vi "State Processing Logic.vi"(8 "error in":errorcluster, 9 "State":T1, 10 "Parameter":variant, 11 "User Input":T2 caption="Command") -> (0 "error out":errorcluster, 2 "Feedback":variant caption="Parameter", 3 "State Out":T1 caption="State")   [LabVIEW 2011]
doc: "[Covers: AB3]\n[Covers: AB4]"
uses:
  TypeDefs/UI to CTRL Command.ctl
  TypeDefs/ATM Controller State.ctl
  TypeDefs/Simulated Database Command.ctl
  TypeDefs/User Console Commands.ctl
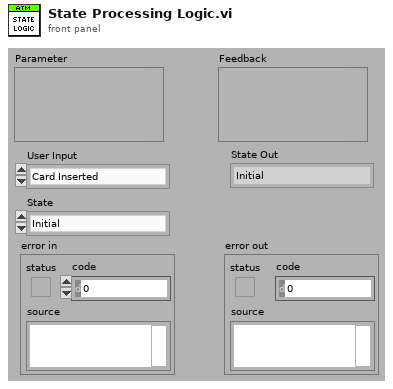
[diagram p1: front panel]
types:
  T1 = typedef "ATM Controller State.ctl" = enum16{"Initial", "Login", "Main Menu", "Balance Inquiry", "Deposit", "Deposit Complete", "Withdrawal", "Withdrawal Success", "Withdrawal Failure", "Terminate", "Lock Out"}
  T2 = typedef "UI to CTRL Command.ctl" = enum16{"Card Inserted", "Keypad Entry", "Button Pressed"}
  T3 = typedef "Simulated Database Command.ctl" = enum16{"Init", "Look up and Lock Account", "Modify Balance", "Get Record", "Commit Record", "Unlock Record", "Close"}
  T4 = typedef "User Console Commands.ctl" = enum16{"Init", "Set ATM Message", "Set ATM Menus", "Disable Controls", "Wait for Input", "Clear Keypad", "Return Card", "Close"}
  T5 = enum16{"Init", "Handle", "Check", "Close", "Set Current Account"}
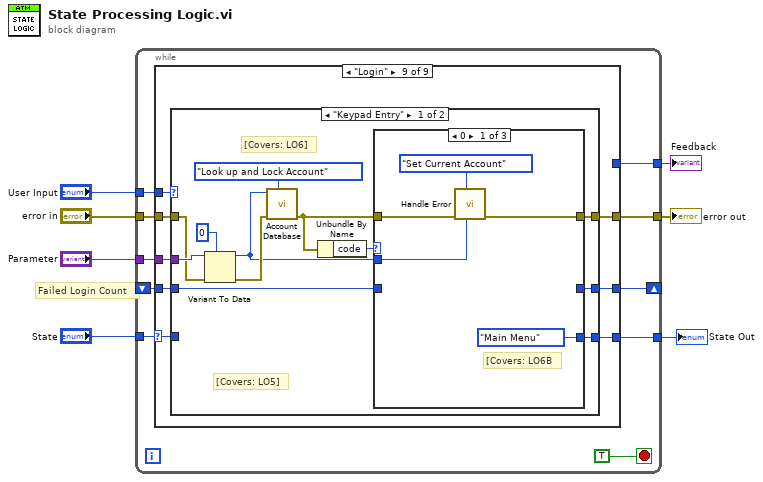
[diagram p0: block diagram]
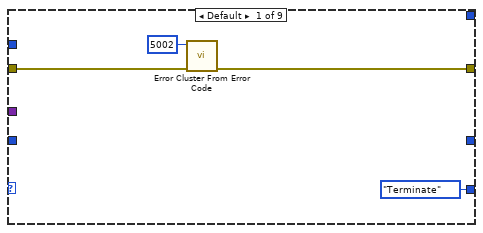
[diagram p2: hidden frame]
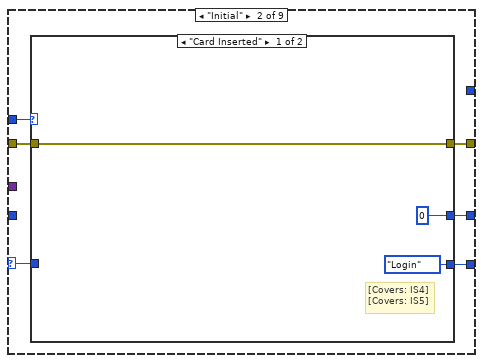
[diagram p3: hidden frame]
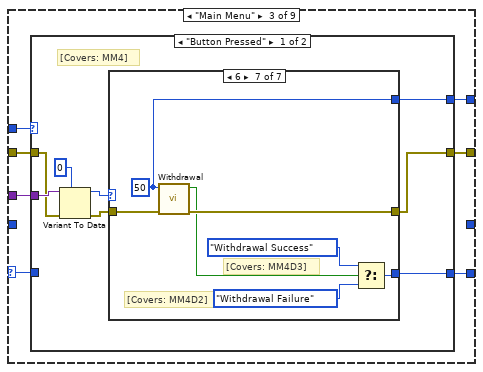
[diagram p5: hidden frame]
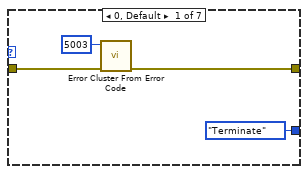
[diagram p6: hidden frame]
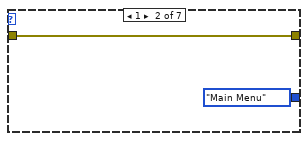
[diagram p7: hidden frame]
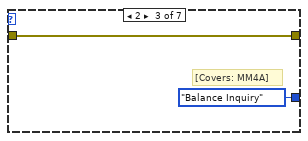
[diagram p8: hidden frame]
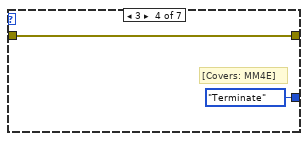
[diagram p9: hidden frame]
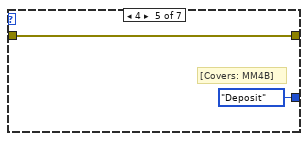
[diagram p10: hidden frame]
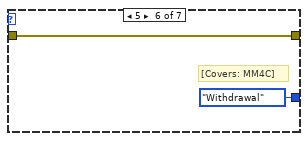
[diagram p11: hidden frame]
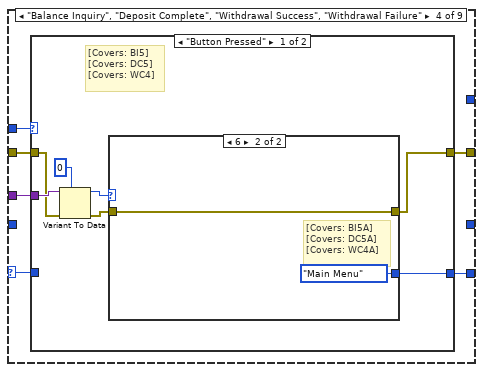
[diagram p13: hidden frame]
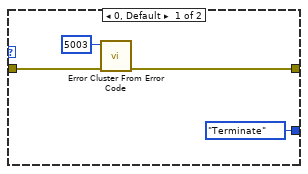
[diagram p14: hidden frame]
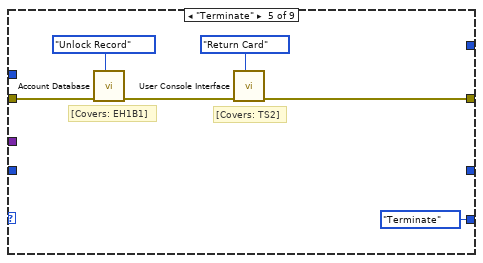
[diagram p16: hidden frame]
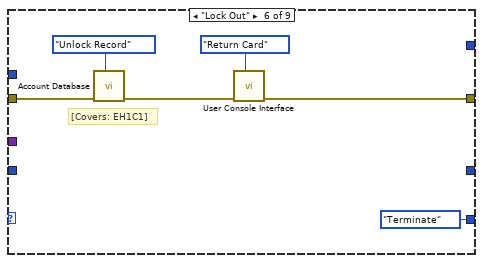
[diagram p17: hidden frame]
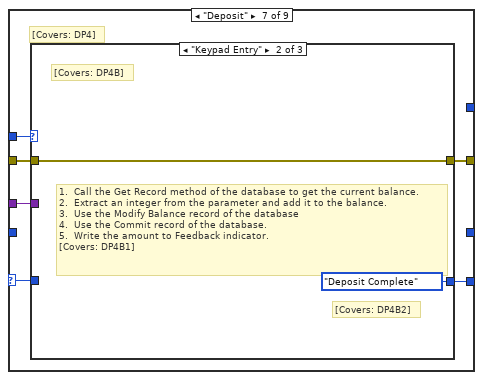
[diagram p18: hidden frame]
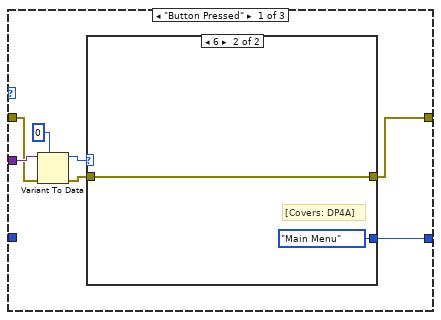
[diagram p19: hidden frame]
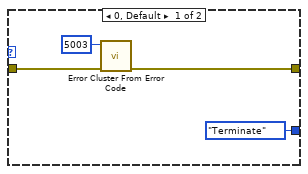
[diagram p20: hidden frame]
diagram:
  # "Failed Login Count"
  n1 = while {
    tunnel: [w17] -> w7
    tunnel: "error in" -> [w16]
    tunnel: "User Input" -> [w15]
    tunnel: "State" -> [w14]
    tunnel: [w13] -> w3
    tunnel: "Parameter" -> [w12]
    shift-right: [w10] -> _
    shift-left: _ -> [w9]
    tunnel: [w8] -> w1
    stop <- TRUE stop-if-true
    n2 = case shown="\"Login\"" w14 {
      selector: w14 -> [_ w23 w35 w72 _ _ w105 w129 w162]
      tunnel: w15 -> [_ w27 w39 w76 _ _ w109 w133 w166]
      tunnel: w16 -> [w20 w26 w38 w75 w94 w100 w108 w132 w165]
      tunnel: [w18 w25 w37 w74 w95 w101 w107 w131 w164] -> w17
      tunnel: [ATM_Controller_State."Terminate" ("State") w24 w36 w73 ATM_Controller_State."Terminate" ("State") ATM_Controller_State."Terminate" ("State") w106 w130 w163] -> w13
      tunnel: w12 -> [_ _ w34 w71 _ _ w104 w128 w161]
      tunnel: [_ w22 _ _ _ _ _ _ w159] -> w10
      tunnel: w9 -> [_ _ _ _ _ _ _ _ w160]
      tunnel: [_ _ w33 _ _ _ _ w127 _] -> w8
      frame Default {
        n3 = call <vilib>:"Error Cluster From Error Code.vi"("error in (no error)"=w20, "error code (0)"=5002) -> ("error out"=w18:errorcluster)  [unwired: 7 in]
      }
      frame "Initial" {
        n4 = case shown="\"Card Inserted\"" w27 {
          tunnel: w26 -> [w29 w32]
          tunnel: [w29 w32] -> w25
          tunnel: [ATM_Controller_State."Login" ("State Out") w31] -> w24
          tunnel: w23 -> [_ w31]
          tunnel: [0 _] -> w22
          frame "Card Inserted" {
            # "[Covers: IS4]\n[Covers: IS5]"
          }
          frame Default {
          }
        }
      }
      frame "Main Menu" {
        n5 = case shown="\"Button Pressed\"" w39 {
          tunnel: w38 -> [w46 w70]
          tunnel: [w42 w70] -> w37
          tunnel: [w41 w69] -> w36
          tunnel: w35 -> [_ w69]
          tunnel: w34 -> [w47 _]
          tunnel: [w40 _] -> w33
          frame "Button Pressed" {
            # "[Covers: MM4]"
            n6 = Variant To Data(error in=w46, type=0 ("index"), Variant=w47) -> (data=w44:i32, error out=w43:errorcluster)
            n7 = case shown="6" w44 {
              tunnel: w43 -> [w51 w53 w55 w57 w59 w61 w68]
              tunnel: [w49 w53 w55 w57 w59 w61 w67] -> w42
              tunnel: [ATM_Controller_State."Terminate" ("State") ATM_Controller_State."Main Menu" ("State") ATM_Controller_State."Balance Inquiry" ("State") ATM_Controller_State."Terminate" ("State") ATM_Controller_State."Deposit" ("State") ATM_Controller_State."Withdrawal" ("State") w63] -> w41
              tunnel: [_ _ _ _ _ _ w62] -> w40
              frame 0, Default {
                n8 = call <vilib>:"Error Cluster From Error Code.vi"("error in (no error)"=w51, "error code (0)"=5003) -> ("error out"=w49:errorcluster)  [unwired: 7 in]
              }
              frame 1 {
              }
              frame 2 {
                # "[Covers: MM4A]"
              }
              frame 3 {
                # "[Covers: MM4E]"
              }
              frame 4 {
                # "[Covers: MM4B]"
              }
              frame 5 {
                # "[Covers: MM4C]"
              }
              frame 6 {
                w62 = 50 ("Amount")
                # "[Covers: MM4D3]"
                # "[Covers: MM4D2]"
                n9 = call "Withdrawal.vi"("error in (no error)"=w68, "Amount"=w62) -> ("error out"=w67:errorcluster, "Successful?"=w66:bool)  [unwired: 8 in]
                n10 = Select(t=ATM_Controller_State."Withdrawal Success" ("State"), s=w66, f=ATM_Controller_State."Withdrawal Failure" ("State")) -> (s? t:f=w63:T1)
              }
            }
          }
          frame Default {
          }
        }
      }
      frame "Balance Inquiry", "Deposit Complete", "Withdrawal Success", "Withdrawal Failure" {
        n11 = case shown="\"Button Pressed\"" w76 {
          tunnel: w75 -> [w82 w91]
          tunnel: [w78 w91] -> w74
          tunnel: [w77 w90] -> w73
          tunnel: w72 -> [_ w90]
          tunnel: w71 -> [w83 _]
          frame "Button Pressed" {
            # "[Covers: BI5]\n[Covers: DC5]\n[Covers: WC4]"
            n12 = Variant To Data(error in=w82, type=0 ("index"), Variant=w83) -> (data=w80:i32, error out=w79:errorcluster)
            n13 = case shown="6" w80 {
              tunnel: w79 -> [w87 w88]
              tunnel: [w85 w88] -> w78
              tunnel: [ATM_Controller_State."Terminate" ("State") ATM_Controller_State."Main Menu" ("State")] -> w77
              frame 0, Default {
                n14 = call <vilib>:"Error Cluster From Error Code.vi"("error in (no error)"=w87, "error code (0)"=5003) -> ("error out"=w85:errorcluster)  [unwired: 7 in]
              }
              frame 6 {
                # "[Covers: BI5A]\n[Covers: DC5A]\n[Covers: WC4A]"
              }
            }
          }
          frame Default {
          }
        }
      }
      frame "Terminate" {
        # "[Covers: EH1B1]"
        # "[Covers: TS2]"
        n15 = call "Account Database.vi"("Command"=Simulated_Database_Command."Unlock Record", "error in (no error)"=w94) -> ("error out"=w93:errorcluster)  [unwired: 7 in, 2 out]
        n16 = call "User Console Interface.vi"("Command"=User_Console_Commands."Return Card", "error in (no error)"=w93) -> ("error out"=w95:errorcluster)  [unwired: 6 in, 3 out]
      }
      frame "Lock Out" {
        # "[Covers: EH1C1]"
        n17 = call "Account Database.vi"("Command"=Simulated_Database_Command."Unlock Record", "error in (no error)"=w100) -> ("error out"=w99:errorcluster)  [unwired: 7 in, 2 out]
        n18 = call "User Console Interface.vi"("Command"=User_Console_Commands."Return Card", "error in (no error)"=w99) -> ("error out"=w101:errorcluster)  [unwired: 6 in, 3 out]
      }
      frame "Deposit" {
        # "[Covers: DP4]"
        n19 = case shown="\"Keypad Entry\"" w109 {
          tunnel: w108 -> [w115 w123 w126]
          tunnel: [w111 w123 w126] -> w107
          tunnel: [w110 ATM_Controller_State."Deposit Complete" ("State") w125] -> w106
          tunnel: w105 -> [_ _ w125]
          tunnel: w104 -> [w116 _ _]
          frame "Button Pressed" {
            n20 = Variant To Data(error in=w115, type=0 ("index"), Variant=w116) -> (data=w113:i32, error out=w112:errorcluster)
            n21 = case shown="6" w113 {
              tunnel: w112 -> [w120 w121]
              tunnel: [w118 w121] -> w111
              tunnel: [ATM_Controller_State."Terminate" ("State") ATM_Controller_State."Main Menu" ("State")] -> w110
              frame 0, Default {
                n22 = call <vilib>:"Error Cluster From Error Code.vi"("error in (no error)"=w120, "error code (0)"=5003) -> ("error out"=w118:errorcluster)  [unwired: 7 in]
              }
              frame 6 {
                # "[Covers: DP4A]"
              }
            }
          }
          frame "Keypad Entry" {
            # "[Covers: DP4B2]"
            # "1.  Call the Get Record method of the database to get the current balance.\n2.  Extract an integer from the parameter and add it to the balance.\n3.  Use the Modify Balance record of the database\n4.  Use the Commit record of the database.\n5.  Write the amount to Feedback indicator.\n[Covers: DP4B1]"
            # "[Covers: DP4B]"
          }
          frame Default {
          }
        }
      }
      frame "Withdrawal" {
        # "[Covers: WD4]"
        n23 = case shown="\"Keypad Entry\"" w133 {
          tunnel: w132 -> [w139 w155 w158]
          tunnel: [w135 w153 w158] -> w131
          tunnel: [w134 w148 w157] -> w130
          tunnel: w129 -> [_ _ w157]
          tunnel: w128 -> [w140 w156 _]
          tunnel: [_ w147 _] -> w127
          frame "Button Pressed" {
            n24 = Variant To Data(error in=w139, type=0 ("index"), Variant=w140) -> (data=w137:i32, error out=w136:errorcluster)
            n25 = case shown="6" w137 {
              tunnel: w136 -> [w144 w145]
              tunnel: [w142 w145] -> w135
              tunnel: [ATM_Controller_State."Terminate" ("State") ATM_Controller_State."Main Menu" ("State")] -> w134
              frame 0, Default {
                n26 = call <vilib>:"Error Cluster From Error Code.vi"("error in (no error)"=w144, "error code (0)"=5003) -> ("error out"=w142:errorcluster)  [unwired: 7 in]
              }
              frame 6 {
                # "[Covers: WD4A]"
              }
            }
          }
          frame "Keypad Entry" {
            # "[Covers: WD4B1B]"
            # "[Covers: WD4B2]"
            # "[Covers: WD4B]"
            n27 = Variant To Data(error in=w155, type=0 ("Amount"), Variant=w156) -> (data=w147:i32, error out=w154:errorcluster)
            n28 = call "Withdrawal.vi"("error in (no error)"=w154, "Amount"=w147) -> ("error out"=w153:errorcluster, "Successful?"=w152:bool)  [unwired: 8 in]
            n29 = Select(t=ATM_Controller_State."Withdrawal Success" ("State"), s=w152, f=ATM_Controller_State."Withdrawal Failure" ("State")) -> (s? t:f=w148:T1)
          }
          frame Default {
          }
        }
      }
      frame "Login" {
        n30 = case shown="\"Keypad Entry\"" w166 {
          tunnel: w165 -> [w171 w199]
          tunnel: [w168 w199] -> w164
          tunnel: [w173 w198] -> w163
          tunnel: w162 -> [_ w198]
          tunnel: w161 -> [w178 _]
          tunnel: w160 -> [w172 _]
          tunnel: [w169 _] -> w159
          frame "Keypad Entry" {
            # "[Covers: LO6]"
            # "[Covers: LO5]"
            n31 = Variant To Data(error in=w171, type=0, Variant=w178) -> (data=w167:i32, error out=w170:errorcluster)
            n32 = call "Account Database.vi"("Command"=Simulated_Database_Command."Look up and Lock Account", "error in (no error)"=w170, "Balance or Account #"=w167) -> ("error out"=w174:errorcluster)  [unwired: 6 in, 2 out]
            n33 = Unbundle By Name(w174) -> ("code"=w175:i32)
            n34 = case shown="0" w175 {
              tunnel: w174 -> [w182 w185 _]
              tunnel: [ATM_Controller_State."Main Menu" ("State") ATM_Controller_State."Terminate" ("State") w191] -> w173
              tunnel: w172 -> [_ _ w197]
              tunnel: [_ _ w196] -> w169
              tunnel: [w181 w185 w187] -> w168
              tunnel: w167 -> [w179 _ _]
              frame 0 {
                # "[Covers: LO6B"
                n35 = call "Handle Error.vi"("Current Account"=w179, "Command"=T5."Set Current Account", "error in (no error)"=w182) -> ("error out"=w181:errorcluster)  [unwired: 6 in, 2 out]
              }
              frame Default {
              }
              frame 5000 {
                # "[Covers: LO6A]\n[Covers: LO6A2]\n[Covers: SC1]"
                # "[Covers: LO6A1]"
                n36 = Increment(x=w197) -> (x+1=w196:i32)
                n37 = call "ATM Message Handler.vi"("Message Name"="Account Verification Failed Message") -> ("error out"=w189:errorcluster, "Message"=w190:string)  [unwired: 9 in]
                n38 = Greater Or Equal?(x=w196, y=3) -> (x >= y?=w194:bool)
                n39 = call "User Console Interface.vi"("Command"=User_Console_Commands."Set ATM Message", "error in (no error)"=w189, "Parameter"=w190) -> ("error out"=w187:errorcluster)  [unwired: 5 in, 3 out]
                n40 = Select(t=ATM_Controller_State."Terminate" ("State"), s=w194, f=ATM_Controller_State."Login" ("State")) -> (s? t:f=w191:T1)
              }
            }
          }
          frame Default {
          }
        }
      }
    }
  }
  "error out" <- w7
  "State Out" <- w3
  "Feedback" <- w1
